vi "3-1 LED Simulator.vi"() -> ()   [LabVIEW 2014]
doc: "------------------------------------\nAuther: Koji Ohashi\nCopyright (c) 2020 Japan LabVIEW Users Group, Volunteer members.\nThis VI is released under the MIT License.\nhttp://opensource.org/licenses/mit-license.php\n------------------------------------"
panel:
  out "LED Status":string
  in  "Maximum Forward Current (mA)":dbl=30.0 min=0.0 step=1.0
  in  "Forward Voltage (V)":dbl=1.6 min=0.0 step=0.1 format="%.1f"
  out "LED":u32(colorbox)
  in  "Power-supply voltage":enum16{"1.8V", "3.3V", "5V"}(ring)=enum."5V"
  in  "Current Limiting\nResistor (ohm)":dbl(knob)=120.0 scale=0.0..1000.0
  out "Current (mA)":dbl format="%#.1f"
  out "Current (A)":dbl format="%#.3f"
  # "LED and\nCurrent Limiting Resistor"
  # "LED Specifications"
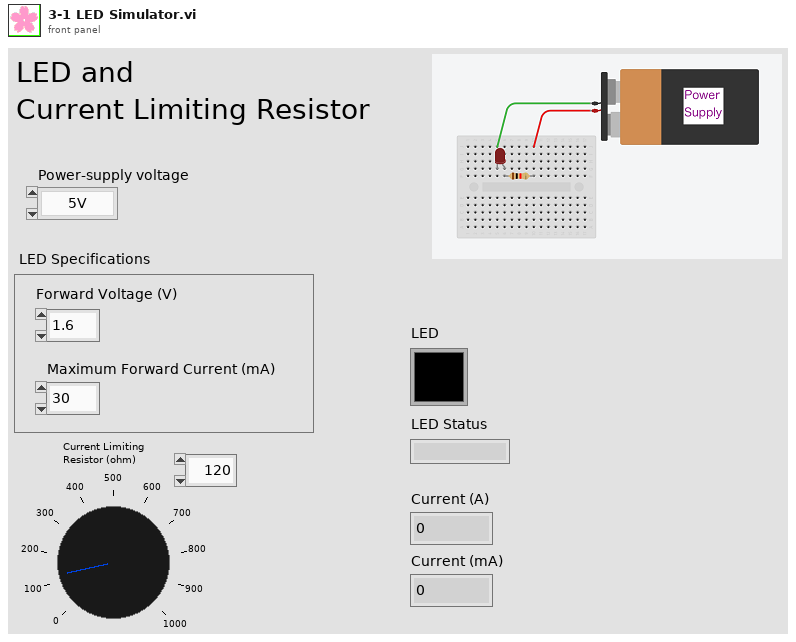
[diagram p1: front panel]
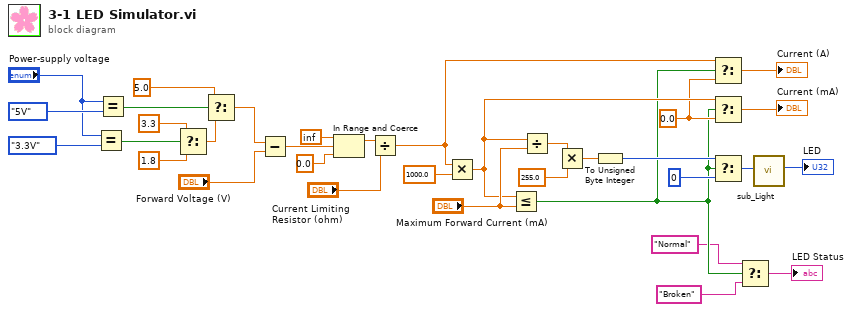
[diagram p0: block diagram]
diagram:
  w9 = 0.0 ("f")
  n1 = Equal?(x="Power-supply voltage", y=enum16{"1.8V", "3.3V", "5V"}."3.3V" ("Enum")) -> (x = y?=w29:bool)
  n2 = Equal?(x="Power-supply voltage", y=enum16{"1.8V", "3.3V", "5V"}."5V" ("Enum")) -> (x = y?=w32:bool)
  n3 = Select(t=3.3 ("電源電圧(V)"), s=w29, f=1.8 ("電源電圧(V)")) -> (s? t:f=w26:dbl)
  n4 = Select(t=5.0 ("電源電圧(V)"), s=w32, f=w26) -> (s? t:f=w22:dbl)
  n5 = Subtract(x=w22, y="Forward Voltage (V)") -> (x-y=w20:dbl)
  n6 = In Range and Coerce(upper limit=inf, x=w20, lower limit=0.0) -> (coerced(x)=w19:dbl)  [unwired: 1 out]
  n7 = Divide(x=w19, y="Current Limiting\nResistor (ohm)") -> (x/y=w13:dbl)
  n8 = Multiply(x=w13, y=1000.0) -> (x*y=w12:dbl)
  n9 = Less Or Equal?(x=w12, y="Maximum Forward Current (mA)") -> (x <= y?=w3:bool)
  n10 = Divide(x=w12, y="Maximum Forward Current (mA)") -> (x/y=w16:dbl)
  n11 = Multiply(x=w16, y=255.0 ("B")) -> (x*y=w14:dbl)
  n12 = To Unsigned Byte Integer(number=w14) -> (unsigned 8bit integer=w5:u8)
  n13 = Select(t=w13, s=w3, f=w9) -> (s? t:f=→"Current (A)":dbl)
  n14 = Select(t=w12, s=w3, f=w9) -> (s? t:f=→"Current (mA)":dbl)
  n15 = Select(t=w5, s=w3, f=u8 0 ("R")) -> (s? t:f=w7:u8)
  n16 = Select(t="Normal", s=w3, f="Broken") -> (s? t:f=→"LED Status":string)
  n17 = call "sub_Light.vi"("Input(0-255)"=w7) -> ("LED"=→"LED":u32)  [unwired: 10 in]
